vi "FTW-Actor-LaunchChildActor-Core.vi"(0 "FTW-ActorInstance In":refnum<class "FTW-ActorInstance.lvclass">, 5 "Actor Instance Configuration":string, 11 "error in":errorcluster) -> (4 "FTW-ActorInstance Out":refnum<class "FTW-ActorInstance.lvclass">, 6 "Initialized Response":string, 8 "Instance Inbox Address":string, 10 "Publishers":cluster{"Name":string, "URI":string}[](array[cluster]), 14 "Identity":string, 15 "error out":errorcluster)   [LabVIEW 2018, in "FTW-ActorInstance.lvclass"]
uses:
  FTW-ActorInstance.lvclass
  Connector/FTW-ActorConnector.lvclass
  d4b2f1f3-3ae1-4726-92fa-5cc5aedbe13b.vi
  JSON/core/FTW-JSON-Core-EncodingFlags.vi
  Reflection/FTW-Reflection-Type.vi
  JSON/FTW-JSON-Parse.vi
  container/FTW-Container-GetFlattenedValue.vi
panel:
  # "Inputs"
  # "Outputs"
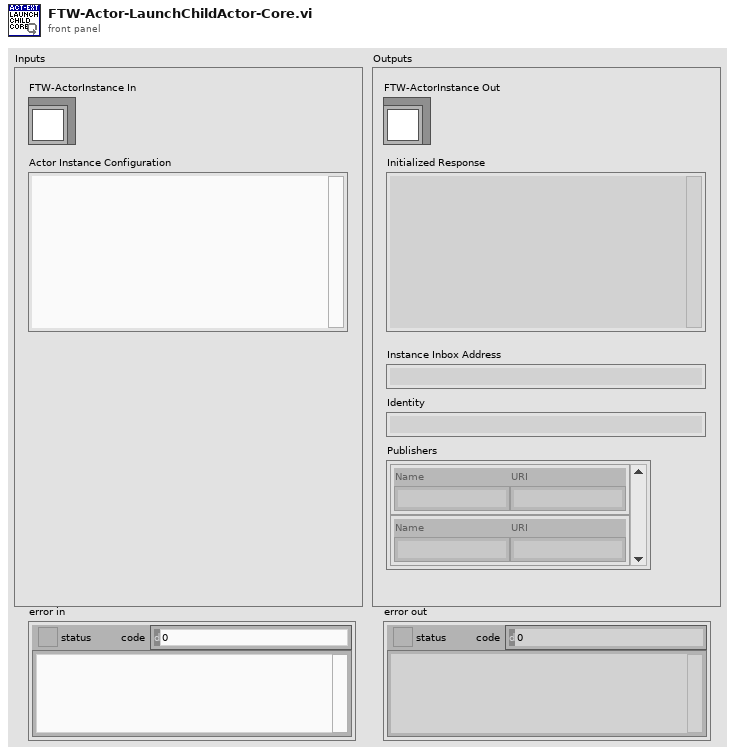
[diagram p1: front panel]
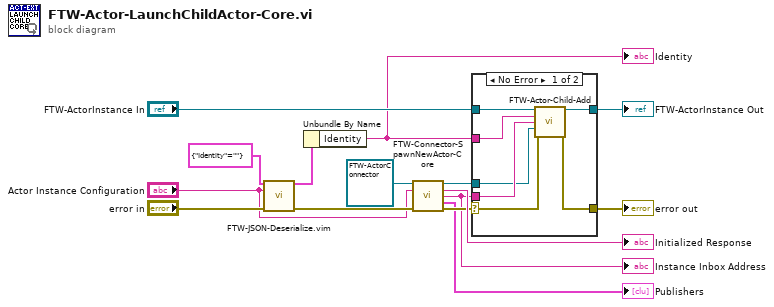
[diagram p0: block diagram]
diagram:
  n1 = call "FTW-JSON-Deserialize.vim"("Type In"=cluster{"Identity":string} {"Identity"=""}, "JSON String"="Actor Instance Configuration", "error in"="error in") -> ("Type Out"=w11:cluster{"Identity":string}, "error out"=w7:errorcluster)  [unwired: 11 in]
  n2 = Unbundle By Name(w11) -> ("Identity"=w2:string)
  "Identity" <- w2
  n3 = call "FTW-Connector-SpawnNewActor-Core.vi"("FTW Actor Connector Type"=refnum<class "FTW-ActorConnector.lvclass"> refnum, "Configuration"="Actor Instance Configuration", "error in"=w7) -> ("FTW Actor Connector"=w3:refnum<class "FTW-ActorConnector.lvclass">, "Initialized Response"=→"Initialized Response":string, "Instance Inbox Address"=w4:string, "Publishers"=→"Publishers":cluster{"Name":string, "URI":string}[], "error out"=w6:errorcluster)  [unwired: 8 in]
  "Instance Inbox Address" <- w4
  n4 = case shown="No Error" w6 {
    selector: w6 -> [w22 w23]
    tunnel: "FTW-ActorInstance In" -> [w20 w24]
    tunnel: [w19 w24] -> w13
    tunnel: [w21 w23] -> w8
    tunnel: w2 -> [w18 _]
    tunnel: w4 -> [w17 _]
    tunnel: w3 -> [w16 _]
    frame No Error {
      n5 = call "FTW-Actor-Child-Add.vi"("FTW-ActorExtended In"=w20, "Identity"=w18, "Inbox Address"=w17, "Connection"=w16, "error in"=w22) -> ("FTW-ActorExtended Out"=w19:refnum<class "FTW-ActorInstance.lvclass">, "error out"=w21:errorcluster)  [unwired: 9 in]
    }
    frame Error {
    }
  }
  "FTW-ActorInstance Out" <- w13
  "error out" <- w8
